vi "Global - Handle V1.vi"() -> ()   [LabVIEW 2019]
panel:
  in  "Handle":refnum<visa-resource-name>[](array[refnum])
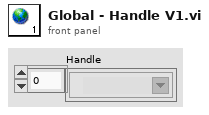
[diagram p1: front panel]
diagram:
